vi "Create DSFTransfer.vi"(8 "error in (no error)":errorcluster, 9 "DSFTransfer info":T1, 10 "id":string, 11 "DSFTransfer in":refnum<class "DSFTransfer.lvclass">) -> (0 "error out":errorcluster, 3 "DSFTransfer out":refnum<class "DSFTransfer.lvclass">)   [LabVIEW 2017, in "DSFTransfer.lvclass"]
uses:
  DSFTransfer.lvclass
  DSFTransfer.lvclass/DSFTransfer.ctl
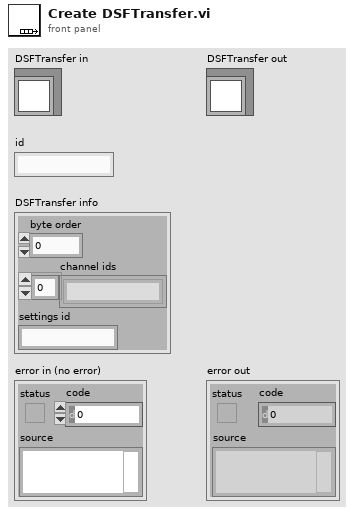
[diagram p1: front panel]
types:
  T1 = cluster{"byte order":i32, "channel ids":string[], "settings id":string}
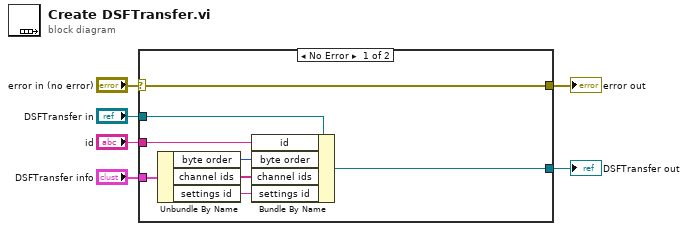
[diagram p0: block diagram]
diagram:
  n1 = case shown="No Error" "error in (no error)" {
    selector: "error in (no error)" -> [w13 w16]
    tunnel: [w13 w16] -> w5
    tunnel: [w12 w15] -> w3
    tunnel: "DSFTransfer in" -> [w14 w15]
    tunnel: "id" -> [w11 _]
    tunnel: "DSFTransfer info" -> [w10 _]
    frame No Error {
      n2 = Unbundle By Name(w10) -> ("byte order"=w9:i32, "channel ids"=w8:string[], "settings id"=w7:string)
      n3 = Bundle By Name(cluster=w14, "id"=w11, "byte order"=w9, "channel ids"=w8, "settings id"=w7) -> (w12:refnum<class "DSFTransfer.lvclass">)
    }
    frame Error {
    }
  }
  "error out" <- w5
  "DSFTransfer out" <- w3
